vi "GEA3 Valve Step Example.vi"() -> ()   [LabVIEW 2016]
uses:
  type defs/Data In.ctl
  library/GEA2_Toolkit.lvlib
panel:
  in  "Disable Check":bool=TRUE
  out "Initial Mix Valve Position":u16
  out "Final Mix Valve Position":u16
  out "GEA Message":T1 {"Command" format="%02x"; "Destination" format="%02x"; "Source" format="%02x"}
  in  "MIX VALVE STEP OFFSET (0x400A)":i16
  out "Raw Data Out":string
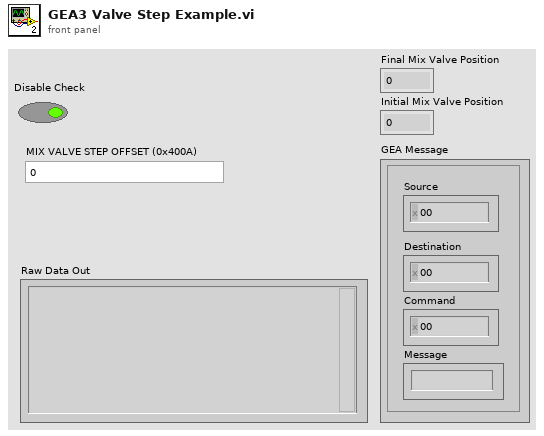
[diagram p1: front panel]
types:
  T1 = typedef "GEA2_Toolkit.lvlib/Data In.ctl" = cluster{"Source":u8, "Destination":u8, "Command":u8, "Message":string}
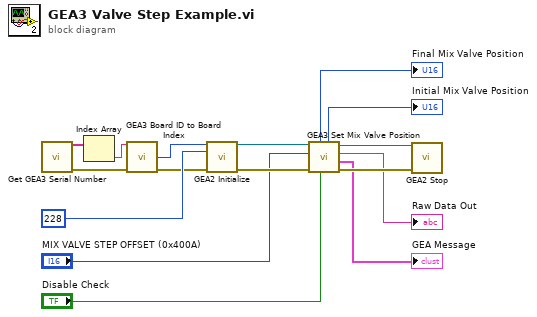
[diagram p0: block diagram]
diagram:
  n1 = call "Get GEA3 Serial Number.vi"() -> ("GEA3 Serial Numbers"=w14:string[], "Error Out"=w13:errorcluster)  [unwired: 14 in]
  n2 = Index Array(array=w14) -> (element=w15:string)  [unwired: 1 in]
  n3 = call "GEA3 Board ID to Board Index.vi"("GEA3 Serial Number"=w15, "Error In"=w13) -> ("Board Index"=w12:i32, "Error Out"=w11:errorcluster)  [unwired: 9 in, 3 out]
  n4 = call "GEA2 Initialize.vi"("Board Index"=w12, "Source Address"=u8 228, "error in"=w11) -> ("GEA2 Reference Out"=w10:refnum<k24>, "error out"=w9:errorcluster)  [unwired: 10 in, 1 out]
  n5 = call "GEA3 Set Mix Valve Position.vi"("Disable Check"="Disable Check", "error in (no error)"=w9, "MIX VALVE STEP OFFSET (0x400A)"="MIX VALVE STEP OFFSET (0x400A)", ".NET Refnum in"=w10) -> ("error out"=w7:errorcluster, "GEA Message"=→"GEA Message":T1, "Raw Data Out"=→"Raw Data Out":string, ".NET Refnum out"=w8:refnum<k24>, "Initial Mix Valve Position"=→"Initial Mix Valve Position":u16, "Final Mix Valve Position"=→"Final Mix Valve Position":u16)  [unwired: 2 in]
  n6 = call "GEA2 Stop.vi"("GEA2 Reference In"=w8, "Error In"=w7) -> ()  [unwired: 13 in, 1 out]
